vi "Instr_InitObject.vi"(8 "error in (no error)":errorcluster, 9 "Instrument Configuration":variant, 10 "GPIB Address":string, 11 "KE3700A in":refnum<class "KE3706A.lvclass">) -> (0 "error out":errorcluster, 3 "KE3700A out":refnum<class "KE3706A.lvclass">)   [LabVIEW 2013, in "KE3706A.lvclass"]
uses:
  KE3706A.lvclass
  KE3706A_CommandsGlobal.vi
  InstrumentSetup.vi
  <instrlib>/Keithley 3706/Keithley 3700 Series.lvlib
  InstrControl.lvclass
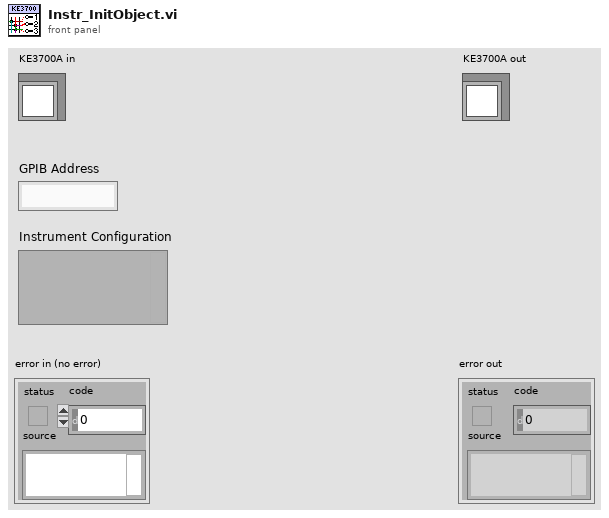
[diagram p1: front panel]
types:
  T1 = cluster{"Mux1 slot":string, "Mux2 slot":string, "KE3706A.lvclass":refnum<class "KE3706A.lvclass">}
  T2 = cluster{"Instrument name":string, "Instrument type":u16, "Command \"Matrix Reset\"":string, "Command \"Connect MUX Channel\"":string, "Command \"Disconnect Matrix Channels\"":string, "Mux1 slot":string, "Mux2 slot":string}
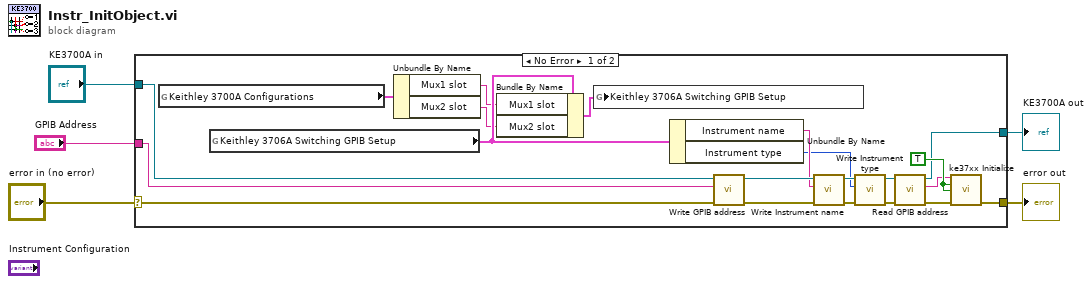
[diagram p0: block diagram]
diagram:
  n1 = case shown="No Error" "error in (no error)" {
    selector: "error in (no error)" -> [w12 w28]
    tunnel: "KE3700A in" -> [w23 w27]
    tunnel: [w6 w28] -> w3
    tunnel: [w9 w27] -> w2
    tunnel: "GPIB Address" -> [w13 _]
    frame No Error {
      w26 = TRUE
      n2 = global read "InstrumentSetup.vi" "Keithley 3700A Configurations"() -> (w18:T1)
      n3 = global read "KE3706A_CommandsGlobal.vi" "Keithley 3706A Switching GPIB Setup"() -> (w17:T2)
      n4 = Unbundle By Name(w18) -> ("Mux1 slot"=w16:string, "Mux2 slot"=w15:string)
      n5 = Bundle By Name(cluster=w17, "Mux1 slot"=w16, "Mux2 slot"=w15) -> (w14:T2)
      n6 = global write "KE3706A_CommandsGlobal.vi" "Keithley 3706A Switching GPIB Setup"(w14) -> ()
      n7 = Unbundle By Name(w17) -> ("Instrument name"=w20:string, "Instrument type"=w19:u16)
      n8 = call-dynamic "Write GPIB address.vi"("error in (no error)"=w12, "GPIB address"=w13, "InstControl in"=w23) -> ("error out"=w25:errorcluster, "InstControl out"=w22:refnum<class "KE3706A.lvclass">)  [unwired: 7 in]
      n9 = call-dynamic "Write Instrument name.vi"("error in (no error)"=w25, "Instrument name"=w20, "InstControl in"=w22) -> ("error out"=w24:errorcluster, "InstControl out"=w21:refnum<class "KE3706A.lvclass">)  [unwired: 7 in]
      n10 = call-dynamic "Write Instrument type.vi"("error in (no error)"=w24, "Instrument type"=w19, "InstControl in"=w21) -> ("error out"=w11:errorcluster, "InstControl out"=w10:refnum<class "KE3706A.lvclass">)  [unwired: 7 in]
      n11 = call-dynamic "Read GPIB address.vi"("error in (no error)"=w11, "InstControl in"=w10) -> ("error out"=w7:errorcluster, "GPIB address"=w8:string, "InstControl out"=w9:refnum<class "KE3706A.lvclass">)  [unwired: 7 in]
      n12 = call <instrlib>:"ke37xx Initialize.vi"("VISA resource name"=w8, "ID Query? (T: Yes)"=w26, "Reset? (T: Yes)"=w26, "error in (no error)"=w7) -> ("error out"=w6:errorcluster)  [unwired: 10 in, 1 out]
    }
    frame Error {
    }
  }
  "error out" <- w3
  "KE3700A out" <- w2
